vi "Disabled.vi"(7 "Robot Mode":T2, 10 "Match Info":T1={"Autonomous Elapsed Seconds"=0.0, "TeleOp Elapsed Seconds"=0.0, "Disabled Elapsed Seconds"=0.0, "Visited Autonomous"=FALSE, "Visited TeleOp"=FALSE, "Visited Disabled"=FALSE, "Autonomous Settings"={"Autonomous Style"=enum."Independent", "VI Refnum"=refnum}}, 11 "Call Context":T3) -> ()   [LabVIEW 2017]
doc: "This VI is called each time a disabled packet is received from the DS. It can be used to prepare for the next robot mode, to calibrate sensors, etc."
uses:
  <vilib>/Rock Robotics/WPI/DriverStation/WPI_DriverStationDerivedRobotMode.ctl
  <vilib>/Rock Robotics/WPI/DriverStation/WPI_DriverStationRobotMode2.ctl
  <vilib>/Rock Robotics/WPI/DriverStation/WPI_DriverStationMatch Info.ctl
  <vilib>/Rock Robotics/Network Tables/NT Read String.vi
  <vilib>/Rock Robotics/Network Tables/NT Write String Array.vi
  Auton/Command Parser/Active Command.vi
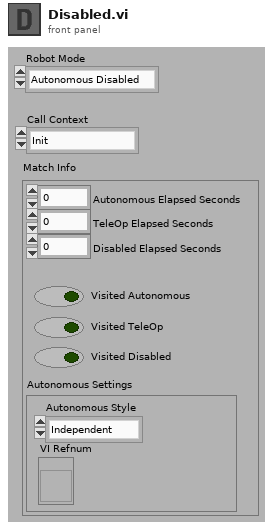
[diagram p1: front panel]
types:
  T1 = typedef "WPI_DriverStationMatch Info.ctl" = cluster{"Autonomous Elapsed Seconds":dbl, "TeleOp Elapsed Seconds":dbl, "Disabled Elapsed Seconds":dbl, "Visited Autonomous":bool, "Visited TeleOp":bool, "Visited Disabled":bool, "Autonomous Settings":cluster{"Autonomous Style":enum16{"Iterative", "Independent"}, "VI Refnum":refnum<vi>}}
  T2 = typedef "WPI_DriverStationRobotMode2.ctl" = enum16{"Autonomous Disabled", "Autonomous Enabled", "Teleop Disabled", "Teleop Enabled", "Disconnected", "Finish", "Test Disabled", "Test Enabled", "Emergency Stopped"}
  T3 = typedef "WPI_DriverStationDerivedRobotMode.ctl" = enum16{"Init", "Execute", "Stop"}
  T4 = typedef "Single Sequence.ctl" = cluster{"Sequence Array":T5[]}
  T5 = typedef "Sequence Command.ctl" = cluster{"Sequence Name":string, "Plate Arrangement":T6, "Command Name":string, "Data":variant, "Sequence Number":u32}
  T6 = typedef "Plate Arrangement.ctl" = cluster{"LR*":bool, "LL*":bool, "RL*":bool, "RR*":bool}
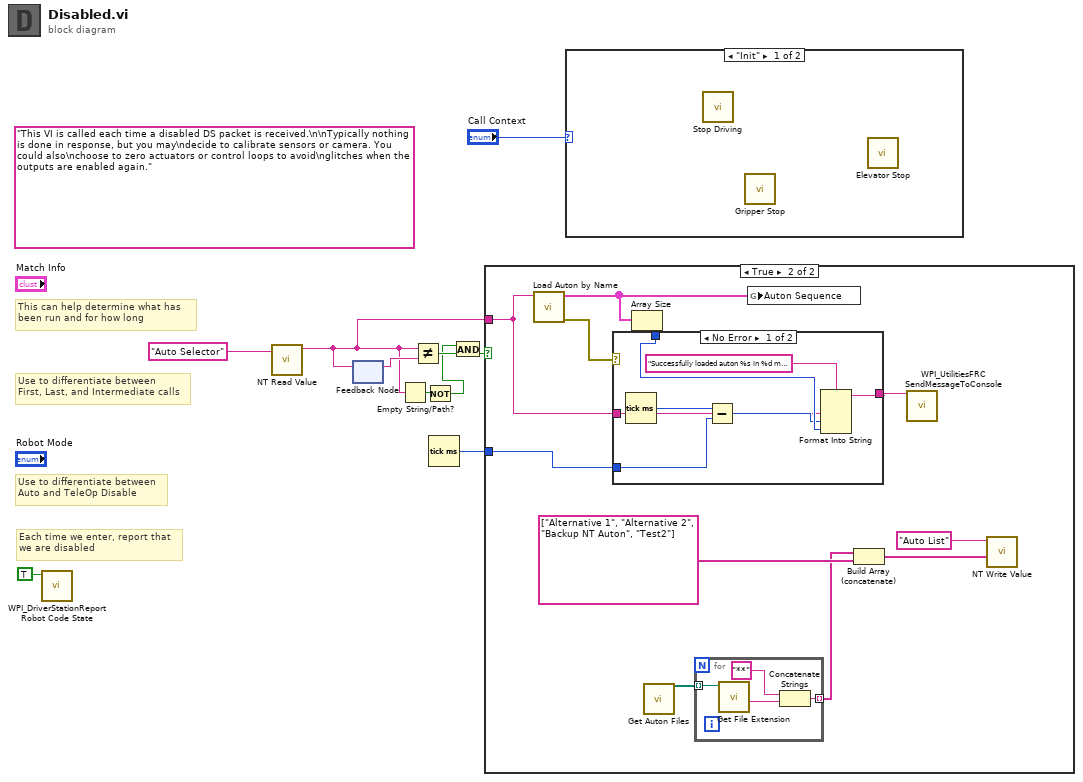
[diagram p0: block diagram]
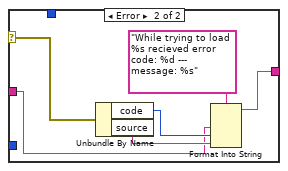
[diagram p4: hidden frame]
diagram:
  (unwired) "This VI is called each time a disabled DS packet is received.\n\nTypically nothing is done in response, but you may\ndecide to calibrate sensors or camera. You could also\nchoose to zero actuators or control loops to avoid\nglitches when the outputs are enabled again."
  # "Each time we enter, report that\nwe are disabled"
  # "Use to differentiate between\nFirst, Last, and Intermediate calls"
  # "This can help determine what has\nbeen run and for how long"
  # "Use to differentiate between\nAuto and TeleOp Disable"
  n1 = call <vilib>:"WPI_DriverStationReport Robot Code State.vi"("Disabled"=TRUE ("Autonomous")) -> ()  [unwired: 10 in, 1 out]
  n2 = call-poly <vilib>:"NT Read Value.vi"("Name"="Auto Selector") -> ("String"=w4:string)  [unwired: 9 in, 1 out]
  n3 = feedback-in #1(w4) -> ()
  n4 = feedback #1() -> (w8:string)  [unwired: 1 in]
  n5 = Empty String/Path?(string/path=w4) -> (empty?=w3:bool)
  n6 = Not Equal?(x=w4, y=w8) -> (x != y?=w7:bool)
  n7 = Not(x=w3) -> (.not. x?=w2:bool)
  n8 = Tick Count (ms)() -> (millisecond timer value=w6:u32)
  n9 = And(x=w2, y=w7) -> (x .and. y?=w5:bool)
  n10 = case shown="True" w5 {
    tunnel: w6 -> [_ w20]
    tunnel: w4 -> [_ w17]
    frame False {
    }
    frame True {
      n11 = call "Load Auton by Name.vi"("String"=w17) -> ("error out"=w21:errorcluster, "Auton Sequence"=w19:T4[])  [unwired: 9 in]
      n12 = Array Size(array=w19) -> (size(s)=w18:i32)
      n13 = case shown="No Error" w21 {
        selector: w21 -> [_ w38]
        tunnel: w20 -> [w31 _]
        tunnel: w18 -> [w29 _]
        tunnel: w17 -> [w27 w34]
        tunnel: [w26 w33] -> w16
        frame No Error {
          n14 = Tick Count (ms)() -> (millisecond timer value=w32:u32)
          n15 = Subtract(x=w32, y=w31) -> (x-y=w28:u32)
          n16 = Format Into String(format string="Successfully loaded auton %s in %d ms with %d sequences.", w27, w28, w29) -> (resulting string=w26:string)  [unwired: 2 in, 1 out]
        }
        frame Error {
          n17 = Unbundle By Name(w38) -> ("code"=w36:i32, "source"=w35:string)
          n18 = Format Into String(format string="While trying to load %s recieved error code: %d --- message: %s", w34, w36, w35) -> (resulting string=w33:string)  [unwired: 2 in, 1 out]
        }
      }
      n19 = call "Get Auton Files.vi"() -> ("All Files in Dir"=w13:path[])  [unwired: 11 in]
      n20 = for {
        tunnel: w13 -> [w25] mode=indexing
        tunnel: [w22] -> w12 mode=indexing
        n21 = call <vilib>:"Get File Extension.vi"("file"=w25) -> ("filename without extension"=w24:string)  [unwired: 6 in, 4 out]
        n22 = Concatenate Strings("**" ("string"), w24) -> (w22:string)
      }
      n23 = global write "Active Command.vi" "Auton Sequence"(w19) -> ()
      n24 = Build Array (concatenate)(w12, string[] ["Alternative 1", "Alternative 2", "Backup NT Auton", "Test2"] ("String Array")) -> (w11:string[])
      n25 = call <vilib>:"WPI_UtilitiesFRC SendMessageToConsole.vi"("Message"=w16) -> ()  [unwired: 14 in, 1 out]
      n26 = call-poly <vilib>:"NT Write Value.vi"("String Array"=w11, "Name"="Auto List") -> ()  [unwired: 9 in, 1 out]
    }
  }
  n27 = case shown="\"Init\"" "Call Context" {
    frame "Init" {
      n28 = call "Stop Driving.vi"() -> ()  [unwired: 11 in, 1 out]
      n29 = call "Gripper Stop.vi"() -> ()  [unwired: 11 in, 1 out]
      n30 = call "Elevator Stop.vi"() -> ()  [unwired: 11 in, 1 out]
    }
    frame "Execute", Default {
    }
  }
